vi "Process.vi"(8 "error in (no error)":errorcluster, 11 "DebuggingTerminal":refnum<class "DebuggingTerminal.lvclass">) -> ()   [LabVIEW 2013, in "MQTT Base.lvlib" / "DebuggingTerminal.lvclass"]
uses:
  DebuggingTerminal.lvclass
  Packet Arrival -- cluster.ctl
  <vilib>/LabVIEW Open Source Project/MQTT Control Packets/Control Packets/ControlPacket/ControlPacket.lvclass
  DebuggingTerminal.lvclass/DebuggingTerminal.ctl
  <vilib>/LabVIEW Open Source Project/MQTT Control Packets/Control Packets/ControlPacket/ControlPacket.lvclass/ControlPacket.ctl
  <vilib>/LabVIEW Open Source Project/MQTT Control Packets/Control Packets/MQTT_311/MQTTVersion.lvclass
  <vilib>/LabVIEW Open Source Project/Advanced Structures/Circular Buffers/VariantBuffer/VariantBuffer.lvclass
  <vilib>/LabVIEW Open Source Project/Advanced Structures/Circular Buffers/VariantBufferMap/VariantBufferMap.lvclass
panel:
  in  "auto-scroll IN":bool=TRUE caption="auto-scroll"
  out "Incoming":string
  in  "auto-scroll OUT":bool=TRUE caption="auto-scroll"
  out "Outgoing":string
  # "Incoming"
  # "Outgoing"
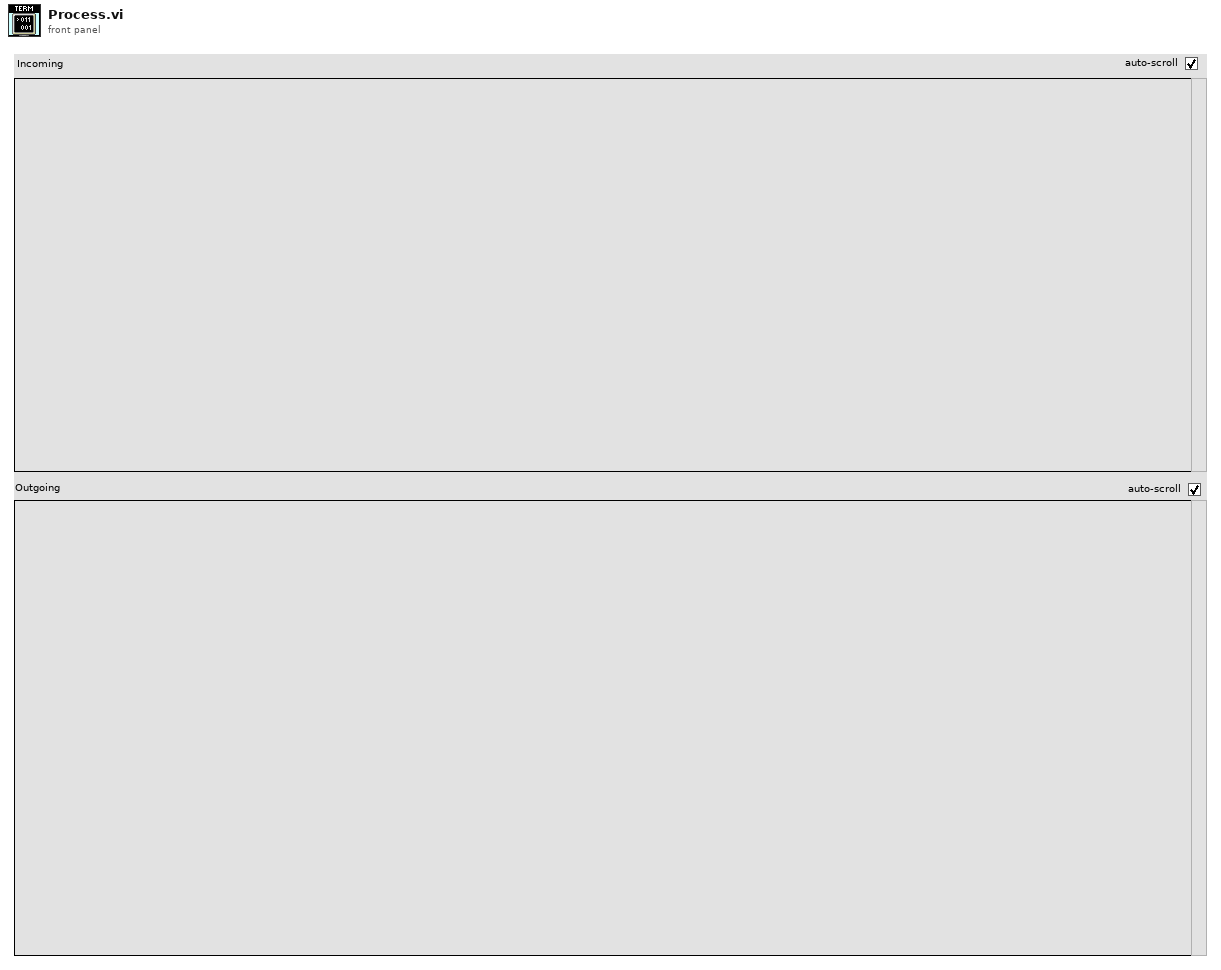
[diagram p1: front panel]
types:
  T1 = typedef "MQTT Base.lvlib/DebuggingTerminal.lvclass/Packet Arrival -- cluster.ctl" = cluster{"Timestamp":timestamp, "Packet":refnum<class "ControlPacket.lvclass">, "Session ID":i32, "outgoing":bool}
  T2 = typedef "MQTT_Control_Packets.lvlib/ControlPacket.lvclass/Control Packet Type -- enum.ctl" = enum16{"Reserved", "CONNECT", "CONNACK", "PUBLISH", "PUBACK", "PUBREC", "PUBREL", "PUBCOMP", "SUBSCRIBE", "SUBACK", "UNSUBSCRIBE", "UNSUBACK", "PINGREQ", "PINGRESP", "DISCONNECT", "AUTH"}
  T3 = typedef "MQTT_Control_Packets.lvlib/ControlPacket.lvclass/QualityOfService -- enum.ctl" = enum16{"0 (At Most Once)", "1 (At Least Once)", "2 (Exactly Once)"}
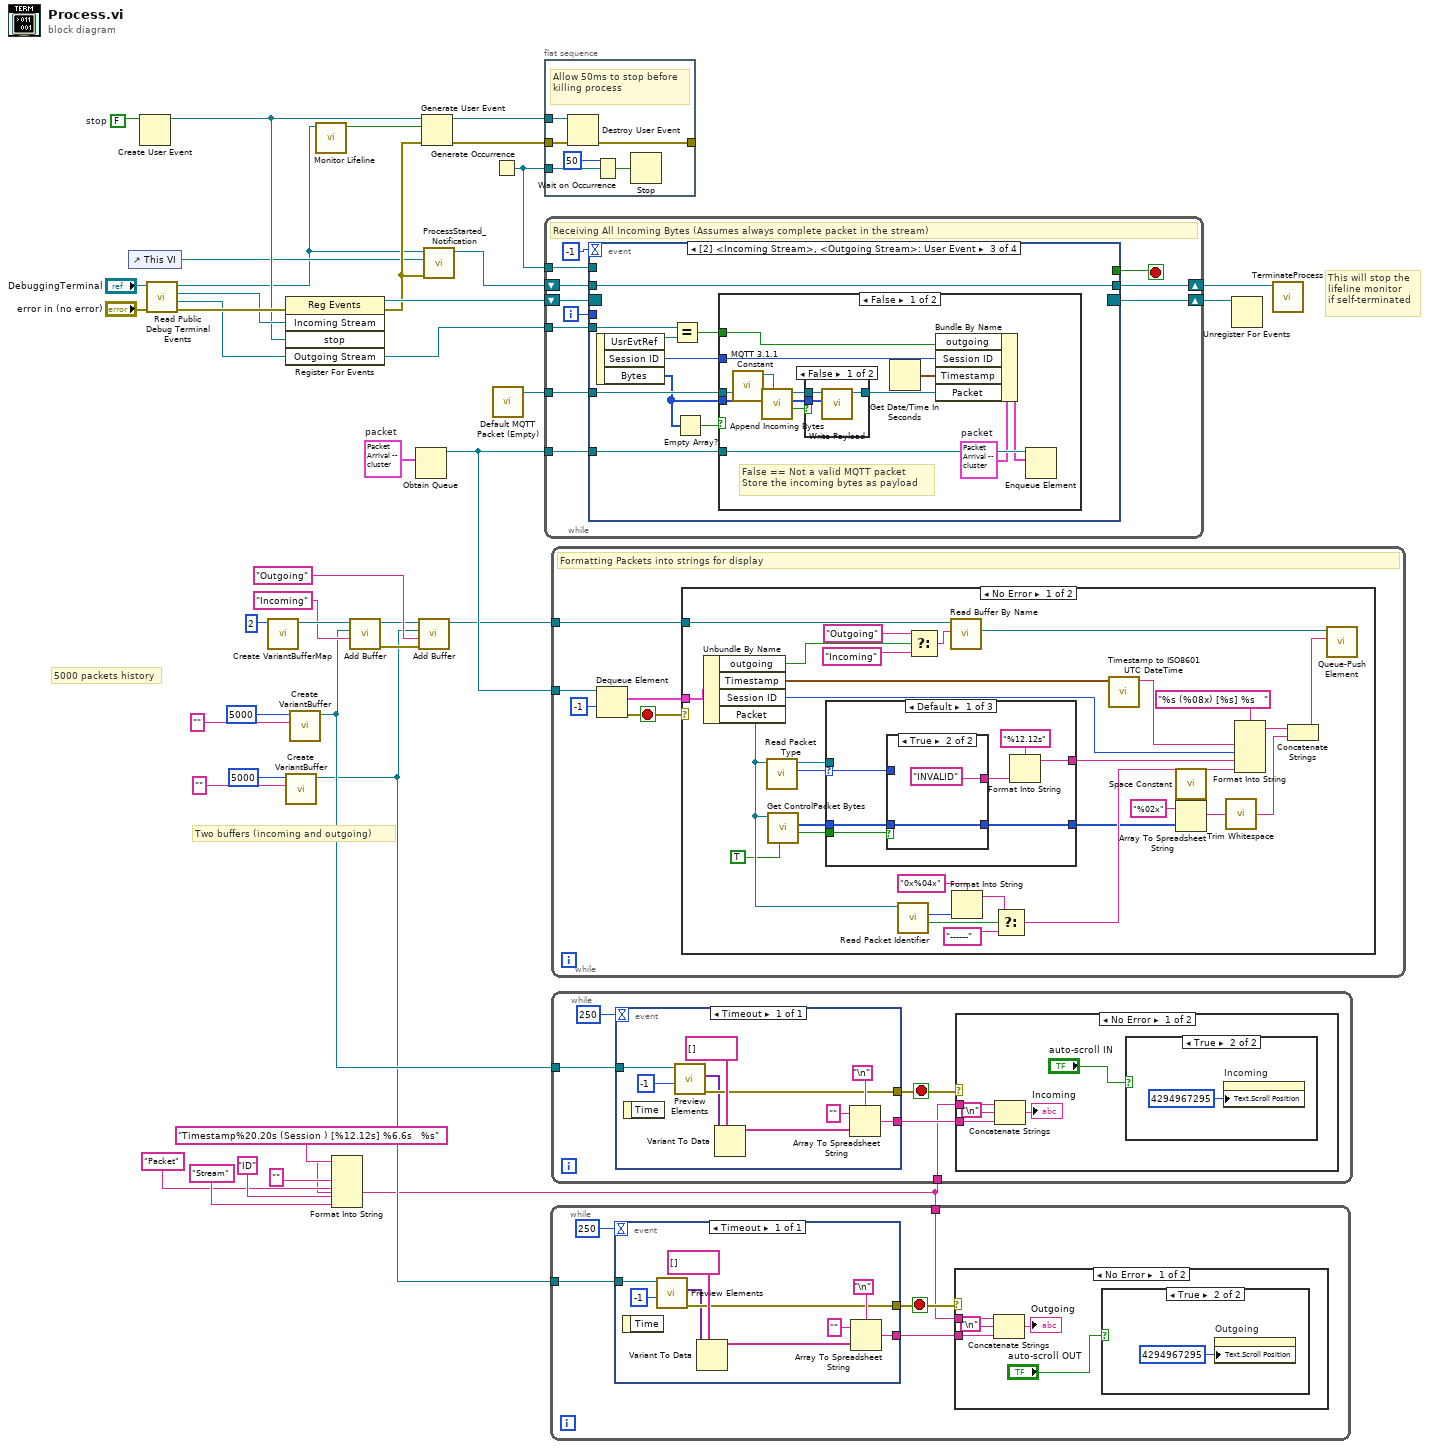
[diagram p0: block diagram]
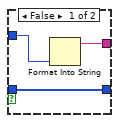
[diagram p6: hidden frame]
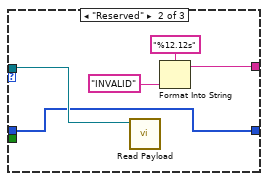
[diagram p7: hidden frame]
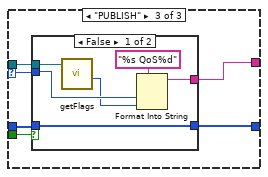
[diagram p8: hidden frame]
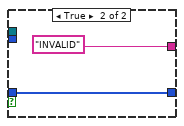
[diagram p9: hidden frame]
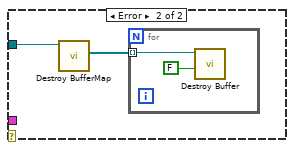
[diagram p10: hidden frame]
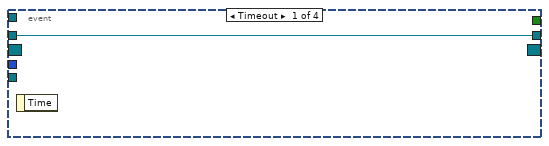
[diagram p11: hidden frame]
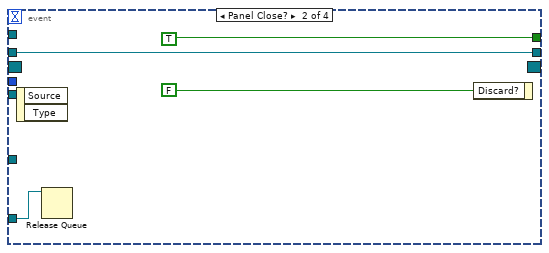
[diagram p12: hidden frame]
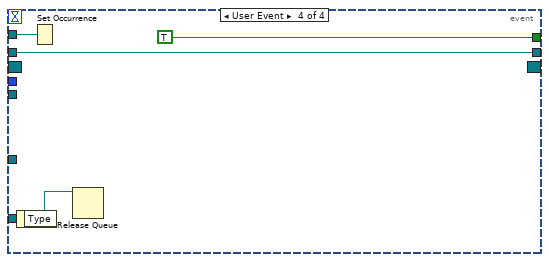
[diagram p15: hidden frame]
diagram:
  w20 = T1 {"Timestamp"=timestamp(0 s since 1904-01-01), "Packet"=refnum, "Session ID"=0, "outgoing"=FALSE}  # packet
  w37 = FALSE  # stop
  # "Two buffers (incoming and outgoing)"
  # "5000 packets history"
  # "This will stop the\nlifeline monitor\nif self-terminated"
  n1 = control-ref of="This VI"() -> (w19:refnum<vi>)
  n2 = Create User Event(user event datatype=w37) -> (user event=w35:refnum<user-event>)  [unwired: 1 in, 1 out]
  n3 = call "Read Public Debug Terminal Events.vi"("error in (no error)"="error in (no error)", "DebuggingTerminal in"="DebuggingTerminal") -> ("error out"=w39:errorcluster, "Outgoing Stream"=w17:refnum<user-event>, "Incoming Stream"=w38:refnum<user-event>, "DebuggingTerminal out"=w6:refnum<class "DebuggingTerminal.lvclass">)  [unwired: 6 in]
  n4 = call <vilib>:"Create VariantBufferMap.vi"("bufSize"=2) -> ("BufferMap"=w11:refnum<data-value>)  [unwired: 9 in, 1 out]
  n5 = register-events(error in=w39, w38, w35, w17) -> (reference out=w33:refnum<event-registration>, error out=w27:errorcluster)  [unwired: 1 in]
  n6 = call <vilib>:"Create VariantBuffer.vi"("default"="" ("input 1"), "bufSize"=5000) -> ("Buffer"=w2:refnum<data-value>)  [unwired: 8 in, 1 out]
  n7 = call <vilib>:"Create VariantBuffer.vi"("default"="" ("input 1"), "bufSize"=5000) -> ("Buffer"=w4:refnum<data-value>)  [unwired: 8 in, 1 out]
  n8 = call "Monitor Lifeline.vi"("DebuggingTerminal in"=w6) -> ("Kill Process"=w36:bool)  [unwired: 10 in]
  n9 = Format Into String(format string="Timestamp%20.20s (Session ) [%12.12s] %6.6s   %s", "" ("input 1"), "Packet" ("input 1"), "ID" ("input 1"), "Stream" ("input 1")) -> (resulting string=w1:string)  [unwired: 2 in, 1 out]
  n10 = call <vilib>:"Add Buffer.vi"("Name"="Incoming" ("input 1"), "Buffer"=w4, "BufferMap in"=w11) -> ("error out"=w8:errorcluster, "BufferMap"=w7:refnum<data-value>)  [unwired: 7 in]
  n11 = Obtain Queue(element data type=w20) -> (queue out=w18:refnum<queue>)  [unwired: 4 in, 2 out]
  n12 = call <vilib>:"Add Buffer.vi"("error in"=w8, "Name"="Outgoing" ("input 1"), "Buffer"=w2, "BufferMap in"=w7) -> ("BufferMap"=w3:refnum<data-value>)  [unwired: 6 in, 1 out]
  n13 = Generate User Event(user event=w35, event data cluster=w36, error in=w27) -> (user event out=w34:refnum<user-event>, error out=w28:errorcluster)  [unwired: 1 in]
  n14 = call "ProcessStarted_Notification.vi"("error in (no error)"=w27, "This VI"=w19, "DebuggingTerminal in"=w6) -> ("DebuggingTerminal out"=w5:refnum<class "DebuggingTerminal.lvclass">)  [unwired: 7 in, 1 out]
  n15 = Generate Occurrence() -> (w32:refnum<k4>)
  n16 = call <vilib>:"Default MQTT Packet (Empty).vi"() -> ("No Packet"=w21:refnum<class "ControlPacket.lvclass">)  [unwired: 11 in]
  n17 = flat-sequence {
    tunnel: w34 -> [w46]
    tunnel: w32 -> [w43]
    tunnel: w28 -> [w42]
    tunnel: [w41] -> _
    frame #0 {
      # "Allow 50ms to stop before killing process"
      n18 = Destroy User Event(user event=w46, error in=w42) -> (error out=w41:errorcluster)
      n19 = Wait on Occurrence(2:w43, 3:50 ("ms timeout (-1)")) -> (0:w44:bool)  [unwired: 1 in]
      n20 = Stop(stop? (T)=w44) -> ()
    }
  }
  n21 = while {
    tunnel: w32 -> [w56]
    shift-right: [w54] -> w31
    shift-left: w33 -> [w57]
    shift-right: [w51] -> w29
    shift-left: w5 -> [w52]
    tunnel: w18 -> [w50]
    tunnel: w21 -> [w49]
    tunnel: w17 -> [w47]
    i -> [w48]
    stop <- w53 stop-if-true
    # "Receiving All Incoming Bytes (Assumes always complete packet in the stream)"
    n22 = event shown="[2] <Incoming Stream>, <Outgoing Stream>: User Event" {
      selector: w57 -> [_ _ _ _]
      dyn-events: [_ _ _ _] -> w54
      timeout: -1 -> [_ _ _ _]
      tunnel: w56 -> [_ _ _ w92]
      tunnel: [_ TRUE ("Discard?") _ TRUE] -> w53
      tunnel: w52 -> [w58 w62 w71 w90]
      tunnel: [w58 w62 w71 w90] -> w51
      tunnel: w50 -> [_ w59 w70 w89]
      tunnel: w49 -> [_ _ w68 _]
      tunnel: w48 -> [_ _ _ _]
      tunnel: w47 -> [_ _ w64 _]
      event Timeout {
        n23 = event-data() -> ()  [unwired: 1 in, 1 out]
      }
      event Panel Close? {
        n24 = event-data() -> ()  [unwired: 1 in, 2 out]
        n25 = Release Queue(queue=w59) -> ()  [unwired: 2 in, 3 out]
        n26 = event-data("Discard?"=FALSE) -> ()  [unwired: 1 in, 1 out]
      }
      event User Event {
        n27 = event-data() -> ("UsrEvtRef"=w65:refnum<user-event>, "Session ID"=w69:i32, "Bytes"=w67:u8[])  [unwired: 1 in]
        n28 = Equal?(x=w64, y=w65) -> (x = y?=w63:bool)
        n29 = Empty Array?(array=w67) -> (empty?=w66:bool)
        n30 = case shown="False" w66 {
          tunnel: w70 -> [w83 _]
          tunnel: w69 -> [w82 _]
          tunnel: w68 -> [w81 _]
          tunnel: w67 -> [w73 _]
          tunnel: w63 -> [w72 _]
          frame False {
            w78 = T1 {"Timestamp"=timestamp(0 s since 1904-01-01), "Packet"=refnum, "Session ID"=0, "outgoing"=FALSE}  # packet
            # "False == Not a valid MQTT packet\nStore the incoming bytes as payload"
            n31 = call <vilib>:"MQTT 3.1.1 Constant.vi"() -> ("MQTT 3.1.1"=w84:refnum<class "MQTTVersion.lvclass">)  [unwired: 11 in]
            n32 = call <vilib>:"Append Incoming Bytes.vi"("MQTT Version (3.1.1)"=w84, "Incoming Packets"=w73, "Incomplete ControlPacket"=w81) -> ("Complete Packet"=w77:bool, "Remaining Packets"=w74:u8[], "ControlPacket"=w75:refnum<class "ControlPacket.lvclass">)  [unwired: 5 in, 1 out]
            n33 = case shown="False" w77 {
              tunnel: [w86 w88] -> w76
              tunnel: w75 -> [w87 w88]
              tunnel: w74 -> [w85 _]
              frame False {
                n34 = call <vilib>:"Write Payload.vi"("Payload"=w85, "ControlPacket in"=w87) -> ("ControlPacket out"=w86:refnum<class "ControlPacket.lvclass">)  [unwired: 9 in]
              }
              frame True {
              }
            }
            n35 = Get Date/Time In Seconds() -> (seconds since 1Jan1904=w79:timestamp)
            n36 = Bundle By Name(cluster=w78, "outgoing"=w72, "Session ID"=w82, "Timestamp"=w79, "Packet"=w76) -> (w80:T1)
            n37 = Enqueue Element(queue=w83, element=w80) -> ()  [unwired: 2 in, 3 out]
          }
          frame True {
          }
        }
      }
      event User Event {
        n38 = event-data() -> ()  [unwired: 1 in, 1 out]
        n39 = Set Occurrence(w92) -> ()
        n40 = Release Queue(queue=w89) -> ()  [unwired: 2 in, 3 out]
      }
    }
  }
  n41 = while {
    tunnel: w2 -> [w94]
    tunnel: w1 -> [w93]
    stop <- w95 stop-if-true
    n42 = event shown="[0] Timeout" {
      selector: _ -> [_]
      dyn-events: _ -> [_]
      timeout: 250 -> [_]
      tunnel: [w107] -> w95
      tunnel: [w108] -> w96
      tunnel: w94 -> [w105]
      event Timeout {
        n43 = event-data() -> ()  [unwired: 1 in, 1 out]
        n44 = call <vilib>:"Preview Elements.vi"("count (-1: all)"=-1, "ByteBuffer in"=w105) -> ("error out"=w107:errorcluster, "elements"=w106:variant[])  [unwired: 7 in, 1 out]
        n45 = Variant To Data(type=string[] [], Variant=w106) -> (data=w111:string[])  [unwired: 1 in, 1 out]
        n46 = Array To Spreadsheet String(delimiter (Tab)="\n", array=w111, 3:"" ("format string")) -> (spreadsheet string=w108:string)
      }
    }
    n47 = case shown="No Error" w95 {
      tunnel: w96 -> [w101 _]
      tunnel: w93 -> [w100 _]
      frame No Error {
        n48 = Concatenate Strings(w100, "\n", w101) -> (→"Outgoing":string)
        n49 = case shown="True" "auto-scroll OUT" {
          frame False {
          }
          frame True {
            n50 = property on="Outgoing" class="Str"("Text.Scroll Position"=u32 4294967295) -> ()  [unwired: 2 in, 2 out]
          }
        }
      }
      frame Error {
      }
    }
  }
  n51 = while {
    tunnel: w18 -> [w116]
    tunnel: w3 -> [w114]
    stop <- w117 stop-if-true
    # "Formatting Packets into strings for display"
    n52 = Dequeue Element(queue=w116, timeout in ms (-1)=-1) -> (element=w113:T1, error out=w117:errorcluster)  [unwired: 1 in, 2 out]
    n53 = case shown="No Error" w117 {
      tunnel: w114 -> [w120 w181]
      tunnel: w113 -> [w148 _]
      frame No Error {
        n54 = Unbundle By Name(w148) -> ("outgoing"=w124:bool, "Timestamp"=w131:timestamp, "Session ID"=w147:i32, "Packet"=w129:refnum<class "ControlPacket.lvclass">)
        n55 = call <vilib>:"Read Packet Type.vi"("ControlPacket in"=w129) -> ("Control Packet Type"=w127:T2, "ControlPacket out"=w143:refnum<class "ControlPacket.lvclass">)  [unwired: 9 in]
        n56 = call <vilib>:"Get ControlPacket Bytes.vi"("Validate? (F)"=TRUE, "ControlPacket"=w129) -> ("Packet invalid"=w126:bool, "Bytes Stream"=w128:u8[])  [unwired: 6 in, 2 out]
        n57 = case shown="Default" w127 {
          selector: w127 -> [w149 _ w171]
          tunnel: [w154 w164 w167] -> w142
          tunnel: w143 -> [_ w162 w166]
          tunnel: [w152 w161 w168] -> w130
          tunnel: w128 -> [w151 w161 w170]
          tunnel: w126 -> [w153 _ w169]
          frame Default {
            n58 = case shown="True" w153 {
              tunnel: [w158 w160] -> w152
              tunnel: w151 -> [w158 w160]
              tunnel: [w156 "INVALID" ("format string")] -> w150
              tunnel: w149 -> [w157 _]
              frame False {
                n59 = Format Into String(w157) -> (resulting string=w156:string)  [unwired: 3 in, 1 out]
              }
              frame True {
              }
            }
            n60 = Format Into String(format string="%12.12s", w150) -> (resulting string=w154:string)  [unwired: 2 in, 1 out]
          }
          frame "Reserved" {
            n61 = call <vilib>:"Read Payload.vi"("ControlPacket in"=w162) -> ()  [unwired: 9 in, 2 out]
            n62 = Format Into String(format string="%12.12s", "INVALID" ("format string")) -> (resulting string=w164:string)  [unwired: 2 in, 1 out]
          }
          frame "PUBLISH" {
            n63 = case shown="False" w169 {
              tunnel: [w177 w179] -> w168
              tunnel: w170 -> [w177 w179]
              tunnel: [w175 "INVALID" ("format string")] -> w167
              tunnel: w171 -> [w176 _]
              tunnel: w166 -> [w173 _]
              frame False {
                n64 = call-dynamic "getFlags.vi"("ControlPacket in"=w173) -> ("QoS"=w172:T3)  [unwired: 7 in, 3 out]
                n65 = Format Into String(format string="%s QoS%d", w176, w172) -> (resulting string=w175:string)  [unwired: 2 in, 1 out]
              }
              frame True {
              }
            }
          }
        }
        n66 = call <vilib>:"Read Packet Identifier.vi"("ControlPacket in"=w129) -> ("Has Packet Identifier"=w133:bool, "Packet Identifier"=w135:u16)  [unwired: 8 in, 1 out]
        n67 = Select(t="Outgoing" ("input 1"), s=w124, f="Incoming" ("input 1")) -> (s? t:f=w121:string)
        n68 = call <vilib>:"Read Buffer By Name.vi"("Name"=w121, "BufferMap in"=w120) -> ("Buffer"=w119:refnum<data-value>)  [unwired: 6 in, 3 out]
        n69 = Format Into String(format string="0x%04x", w135) -> (resulting string=w137:string)  [unwired: 2 in, 1 out]
        n70 = Select(t=w137, s=w133, f="------" ("format string")) -> (s? t:f=w132:string)
        n71 = call <vilib>:"Timestamp to ISO8601 UTC DateTime.vi"("Timestamp (now)"=w131) -> ("ISO8601 UTC DateTime"=w146:string)  [unwired: 10 in]
        n72 = call <vilib>:"Space Constant.vi"() -> ("String"=w140:string)
        n73 = Array To Spreadsheet String(delimiter (Tab)=w140, array=w130, 3:"%02x" ("format string")) -> (spreadsheet string=w141:string)
        n74 = call <vilib>:"Trim Whitespace.vi"("string"=w141) -> ("trimmed string"=w138:string)  [unwired: 1 in]
        n75 = Format Into String(format string="%s (%08x) [%s] %s   ", w146, w147, w142, w132) -> (resulting string=w144:string)  [unwired: 2 in, 1 out]
        n76 = Concatenate Strings(w144, w138) -> (w118:string)
        n77 = call <vilib>:"Queue-Push Element.vi"("element"=w118, "Buffer in"=w119) -> ()  [unwired: 5 in, 5 out]
      }
      frame Error {
        n78 = call <vilib>:"Destroy BufferMap.vi"("Buffer"=w181) -> ("buffers"=w180:refnum<data-value>[])  [unwired: 8 in, 2 out]
        n79 = for {
          tunnel: w180 -> [w183] mode=indexing
          n80 = call <vilib>:"Destroy Buffer.vi"("Return Elements (T)"=FALSE, "Buffer"=w183) -> ()  [unwired: 8 in, 2 out]
        }
      }
    }
  }
  n81 = while {
    tunnel: w1 -> [w186]
    tunnel: w4 -> [w184]
    stop <- w185 stop-if-true
    n82 = event shown="[0] Timeout" {
      selector: _ -> [_]
      dyn-events: _ -> [_]
      timeout: 250 -> [_]
      tunnel: [w198] -> w185
      tunnel: [w199] -> w187
      tunnel: w184 -> [w196]
      event Timeout {
        n83 = event-data() -> ()  [unwired: 1 in, 1 out]
        n84 = call <vilib>:"Preview Elements.vi"("count (-1: all)"=-1, "ByteBuffer in"=w196) -> ("error out"=w198:errorcluster, "elements"=w197:variant[])  [unwired: 7 in, 1 out]
        n85 = Variant To Data(type=string[] [], Variant=w197) -> (data=w202:string[])  [unwired: 1 in, 1 out]
        n86 = Array To Spreadsheet String(delimiter (Tab)="\n", array=w202, 3:"" ("format string")) -> (spreadsheet string=w199:string)
      }
    }
    n87 = case shown="No Error" w185 {
      tunnel: w187 -> [w192 _]
      tunnel: w186 -> [w191 _]
      frame No Error {
        n88 = Concatenate Strings(w191, "\n", w192) -> (→"Incoming":string)
        n89 = case shown="True" "auto-scroll IN" {
          frame False {
          }
          frame True {
            n90 = property on="Incoming" class="Str"("Text.Scroll Position"=u32 4294967295) -> ()  [unwired: 2 in, 2 out]
          }
        }
      }
      frame Error {
      }
    }
  }
  n91 = Unregister For Events(event registration refnum=w31) -> ()  [unwired: 1 in, 1 out]
  n92 = call "TerminateProcess.vi"("DebuggingTerminal in"=w29) -> ()  [unwired: 10 in, 1 out]
